vi "DigitalGraph - Colors.vi"(8 "error in (no error)":errorcluster, 10 "Ctl Refnum":refnum<vi>, 11 "Material-Scheme in":refnum<class "Material-Scheme.lvclass">) -> (0 "error out":errorcluster)   [LabVIEW 2026, in "TSC Material Theme.lvlib" / "Material-Scheme.lvclass"]
doc: "Sets the colors of the digital graph.\n\nColor Rules:\n- Frame, Plot BG: surfaceContainerLowest (preserve transparency)\n- Plot Border: surfaceContainerHighest (preserve transparency)\n- X&Y Scale text: onSurface\n- X&Y Scale gridlines: surfaceContainerHigh (preserve transparency)\n- Plots recolored according to surfaceContainerLowest blending and ratio checking\n- Cursors recolored according to surfaceContainerLowest blending and ratio checking\n- Bus recolored according to surfaceContainerLowest blending and ratio checking\n\n<b>Code Developed By:</b> +\nDaniel Coons +\nTechnology Service Corporation +\nwww.tsc.com/atcs"
uses:
  Material-Scheme.lvclass
  Material-Scheme.lvclass/Material-Scheme.ctl
  Material SubVIs/Color to HSL.vi
  Material SubVIs/Color to Luminance.vi
  Material SubVIs/HSL to Color.vi
  Material SubVIs/tsc--RGB to Color.vi
  <vilib>/Utility/colorconv.llb/Color to RGB.vi
  Material SubVIs/Material SubVIs.lvlib
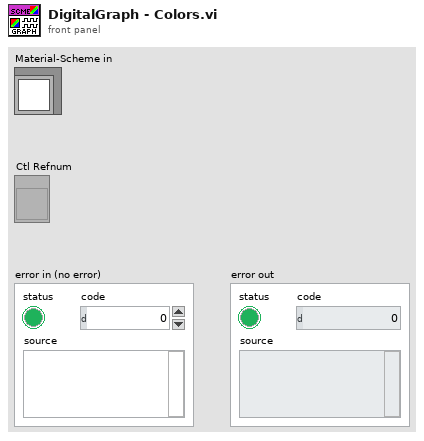
[diagram p1: front panel]
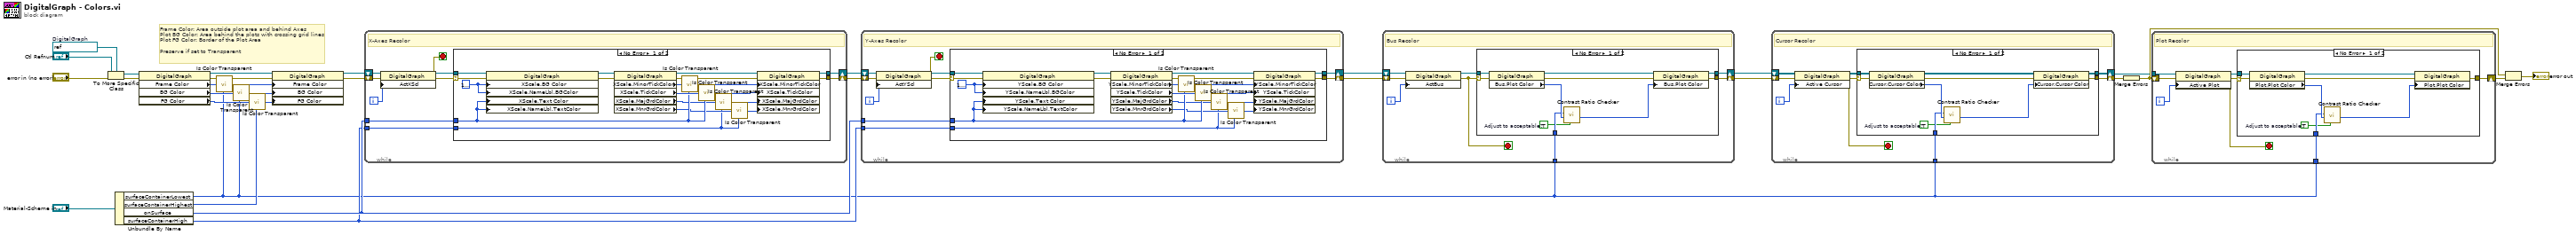
[diagram p0: block diagram]
diagram:
  w29 = refnum<vi> refnum  # DigitalGraph
  # "Frame Color: Area outside plot area and behind Axes\nPlot BG Color: Area behind the plots with crossing grid lines\nPlot FG Color: Border of the Plot Area\n\nPreserve if set to Transparent"
  n1 = To More Specific Class(target class=w29, reference="Ctl Refnum", error in="error in (no error)") -> (specific class reference=w30:refnum<vi>, error out=w31:errorcluster)
  n2 = Unbundle By Name("Material-Scheme in") -> ("surfaceContainerLowest"=w3:u32, "surfaceContainerHighest"=w8:u32, "onSurface"=w15:u32, "surfaceContainerHigh"=w14:u32)
  n3 = property class="DigitalGraph"(reference=w30, error in=w31) -> (reference out=w20:refnum<vi>, error out=w21:errorcluster, "Frame Color"=w10:u32, "BG Color"=w11:u32, "FG Color"=w12:u32)
  n4 = call "Is Color Transparent.vi"("original color"=w10, "desired color"=w3) -> ("updated color"=w9:u32)  [unwired: 3 in]
  n5 = call "Is Color Transparent.vi"("original color"=w11, "desired color"=w3) -> ("updated color"=w13:u32)  [unwired: 3 in]
  n6 = call "Is Color Transparent.vi"("original color"=w12, "desired color"=w8) -> ("updated color"=w22:u32)  [unwired: 3 in]
  n7 = property class="DigitalGraph"(reference=w20, error in=w21, "Frame Color"=w9, "BG Color"=w13, "FG Color"=w22) -> (reference out=w18:refnum<vi>, error out=w19:errorcluster)
  n8 = while {
    shift-right: [w36] -> w17
    shift-left: w19 -> [w40]
    tunnel: w15 -> [w34]
    tunnel: w14 -> [w33]
    shift-right: [w32] -> w16
    shift-left: w18 -> [w39]
    i -> [w38]
    stop <- w37 stop-if-true
    # "X-Axes Recolor"
    n9 = property class="DigitalGraph"(reference=w39, error in=w40, "ActXScl"=w38) -> (reference out=w35:refnum<vi>, error out=w37:errorcluster)
    n10 = case shown="No Error" w37 {
      selector: w37 -> [w59 _]
      tunnel: [w52 _] -> w36
      tunnel: w35 -> [w58 w60]
      tunnel: w34 -> [w48 _]
      tunnel: w33 -> [w42 _]
      tunnel: [w41 w60] -> w32
      frame No Error {
        w57 = u32 16777216 ("X Scale.Name Label.Colors:FG Color")
        n11 = property class="DigitalGraph"(reference=w58, error in=w59, "XScale.BG Color"=w57, "XScale.NameLbl.BGColor"=w57, "XScale.Text Color"=w48, "XScale.NameLbl.TextColor"=w48) -> (reference out=w55:refnum<vi>, error out=w56:errorcluster)
        n12 = property class="DigitalGraph"(reference=w55, error in=w56) -> (reference out=w53:refnum<vi>, error out=w54:errorcluster, "XScale.MinorTickColor"=w51:u32, "XScale.TickColor"=w49:u32, "XScale.MajGrdColor"=w46:u32, "XScale.MnrGrdColor"=w45:u32)
        n13 = call "Is Color Transparent.vi"("original color"=w51, "desired color"=w48) -> ("updated color"=w50:u32)  [unwired: 3 in]
        n14 = call "Is Color Transparent.vi"("original color"=w49, "desired color"=w48) -> ("updated color"=w47:u32)  [unwired: 3 in]
        n15 = call "Is Color Transparent.vi"("original color"=w46, "desired color"=w42) -> ("updated color"=w44:u32)  [unwired: 3 in]
        n16 = call "Is Color Transparent.vi"("original color"=w45, "desired color"=w42) -> ("updated color"=w43:u32)  [unwired: 3 in]
        n17 = property class="DigitalGraph"(reference=w53, error in=w54, "XScale.MinorTickColor"=w50, "XScale.TickColor"=w47, "XScale.MajGrdColor"=w44, "XScale.MnrGrdColor"=w43) -> (reference out=w41:refnum<vi>, error out=w52:errorcluster)
      }
      frame Error {
      }
    }
  }
  n18 = while {
    shift-right: [w65] -> w5
    shift-left: w17 -> [w69]
    tunnel: w15 -> [w63]
    tunnel: w14 -> [w62]
    shift-right: [w61] -> w4
    shift-left: w16 -> [w68]
    i -> [w67]
    stop <- w66 stop-if-true
    # "Y-Axes Recolor"
    n19 = property class="DigitalGraph"(reference=w68, error in=w69, "ActYScl"=w67) -> (reference out=w64:refnum<vi>, error out=w66:errorcluster)
    n20 = case shown="No Error" w66 {
      selector: w66 -> [w88 _]
      tunnel: [w81 _] -> w65
      tunnel: w64 -> [w87 w89]
      tunnel: w63 -> [w77 _]
      tunnel: w62 -> [w71 _]
      tunnel: [w70 w89] -> w61
      frame No Error {
        w86 = u32 16777216 ("X Scale.Name Label.Colors:FG Color")
        n21 = property class="DigitalGraph"(reference=w87, error in=w88, "YScale.BG Color"=w86, "YScale.NameLbl.BGColor"=w86, "YScale.Text Color"=w77, "YScale.NameLbl.TextColor"=w77) -> (reference out=w84:refnum<vi>, error out=w85:errorcluster)
        n22 = property class="DigitalGraph"(reference=w84, error in=w85) -> (reference out=w82:refnum<vi>, error out=w83:errorcluster, "YScale.MinorTickColor"=w80:u32, "YScale.TickColor"=w78:u32, "YScale.MajGrdColor"=w75:u32, "YScale.MnrGrdColor"=w74:u32)
        n23 = call "Is Color Transparent.vi"("original color"=w80, "desired color"=w77) -> ("updated color"=w79:u32)  [unwired: 3 in]
        n24 = call "Is Color Transparent.vi"("original color"=w78, "desired color"=w77) -> ("updated color"=w76:u32)  [unwired: 3 in]
        n25 = call "Is Color Transparent.vi"("original color"=w75, "desired color"=w71) -> ("updated color"=w73:u32)  [unwired: 3 in]
        n26 = call "Is Color Transparent.vi"("original color"=w74, "desired color"=w71) -> ("updated color"=w72:u32)  [unwired: 3 in]
        n27 = property class="DigitalGraph"(reference=w82, error in=w83, "YScale.MinorTickColor"=w79, "YScale.TickColor"=w76, "YScale.MajGrdColor"=w73, "YScale.MnrGrdColor"=w72) -> (reference out=w70:refnum<vi>, error out=w81:errorcluster)
      }
      frame Error {
      }
    }
  }
  n28 = while {
    shift-right: [w95] -> w2
    shift-left: w5 -> [w97]
    tunnel: w3 -> [w92]
    shift-right: [w90] -> w1
    shift-left: w4 -> [w91]
    i -> [w94]
    stop <- w96 stop-if-true
    # "Bus Recolor"
    n29 = property class="DigitalGraph"(reference=w91, error in=w97, "ActBus"=w94) -> (reference out=w93:refnum<vi>, error out=w96:errorcluster)
    n30 = case shown="No Error" w96 {
      selector: w96 -> [w107 _]
      tunnel: [w105 _] -> w95
      tunnel: w93 -> [w104 w108]
      tunnel: w92 -> [w102 _]
      tunnel: [w98 w108] -> w90
      frame No Error {
        w101 = TRUE  # Adjust to acceptable?
        n31 = property class="DigitalGraph"(reference=w104, error in=w107) -> (reference out=w100:refnum<vi>, error out=w106:errorcluster, "Bus.Plot Color"=w103:u32)
        n32 = call "Contrast Ratio Checker.vi"("Adjust to acceptable?"=w101, "On Color"=w103, "Background Color"=w102) -> ("Adjusted Color"=w99:u32)  [unwired: 6 in, 2 out]
        n33 = property class="DigitalGraph"(reference=w100, error in=w106, "Bus.Plot Color"=w99) -> (reference out=w98:refnum<vi>, error out=w105:errorcluster)
      }
      frame Error {
      }
    }
  }
  n34 = while {
    shift-right: [w114] -> w7
    shift-left: w2 -> [w116]
    tunnel: w3 -> [w111]
    shift-right: [w109] -> w6
    shift-left: w1 -> [w110]
    i -> [w113]
    stop <- w115 stop-if-true
    # "Cursor Recolor"
    n35 = property class="DigitalGraph"(reference=w110, error in=w116, "Active Cursor"=w113) -> (reference out=w112:refnum<vi>, error out=w115:errorcluster)
    n36 = case shown="No Error" w115 {
      selector: w115 -> [w126 _]
      tunnel: [w124 _] -> w114
      tunnel: w112 -> [w123 w127]
      tunnel: w111 -> [w121 _]
      tunnel: [w117 w127] -> w109
      frame No Error {
        w120 = TRUE  # Adjust to acceptable?
        n37 = property class="DigitalGraph"(reference=w123, error in=w126) -> (reference out=w119:refnum<vi>, error out=w125:errorcluster, "Cursor.Cursor Color"=w122:u32)
        n38 = call "Contrast Ratio Checker.vi"("Adjust to acceptable?"=w120, "On Color"=w122, "Background Color"=w121) -> ("Adjusted Color"=w118:u32)  [unwired: 6 in, 2 out]
        n39 = property class="DigitalGraph"(reference=w119, error in=w125, "Cursor.Cursor Color"=w118) -> (reference out=w117:refnum<vi>, error out=w124:errorcluster)
      }
      frame Error {
      }
    }
  }
  n40 = Merge Errors(w7) -> (w23:errorcluster)
  n41 = while {
    tunnel: w6 -> [w133]
    shift-right: [w130] -> w25
    shift-left: w23 -> [w134]
    tunnel: w3 -> [w128]
    i -> [w132]
    stop <- w131 stop-if-true
    # "Plot Recolor"
    n42 = property class="DigitalGraph"(reference=w133, error in=w134, "Active Plot"=w132) -> (reference out=w129:refnum<vi>, error out=w131:errorcluster)
    n43 = case shown="No Error" w131 {
      selector: w131 -> [w143 _]
      tunnel: [w137 _] -> w130
      tunnel: w129 -> [w142 _]
      tunnel: w128 -> [w140 _]
      frame No Error {
        w139 = TRUE  # Adjust to acceptable?
        n44 = property class="DigitalGraph"(reference=w142, error in=w143) -> (reference out=w136:refnum<vi>, error out=w138:errorcluster, "Plot.Plot Color"=w141:u32)
        n45 = call "Contrast Ratio Checker.vi"("Adjust to acceptable?"=w139, "On Color"=w141, "Background Color"=w140) -> ("Adjusted Color"=w135:u32)  [unwired: 6 in, 2 out]
        n46 = property class="DigitalGraph"(reference=w136, error in=w138, "Plot.Plot Color"=w135) -> (error out=w137:errorcluster)  [unwired: 1 out]
      }
      frame Error {
      }
    }
  }
  n47 = Merge Errors(w23, w25) -> (→"error out":errorcluster)
